vi "Try Add Sub Object.vi"(8 "error in":errorcluster, 10 "Sub Object":refnum<class "Sub Object.lvclass">, 11 "Object Dictionary in":refnum<class "Object Dictionary.lvclass">) -> (0 "error out":errorcluster, 1 "Success":bool, 3 "Object Dictionary out":refnum<class "Object Dictionary.lvclass">)   [LabVIEW 2020, in "CANopen.lvlib" / "Object Dictionary.lvclass"]
uses:
  Object Dictionary.lvclass
  Sub Object/Sub Object.lvclass
  Object Dictionary.lvclass/Object Dictionary.ctl
  Sub Objects Dictionary/Sub Objects Dictionary.lvclass
  Object Entry/Object Entry.lvclass
  Ordered-Dictionary/Ordered Object Dictionary/Source/Ordered Object Dictionary.lvclass
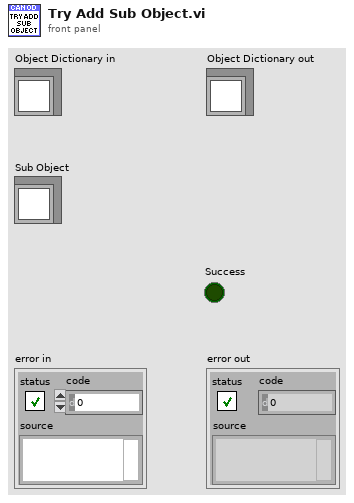
[diagram p1: front panel]
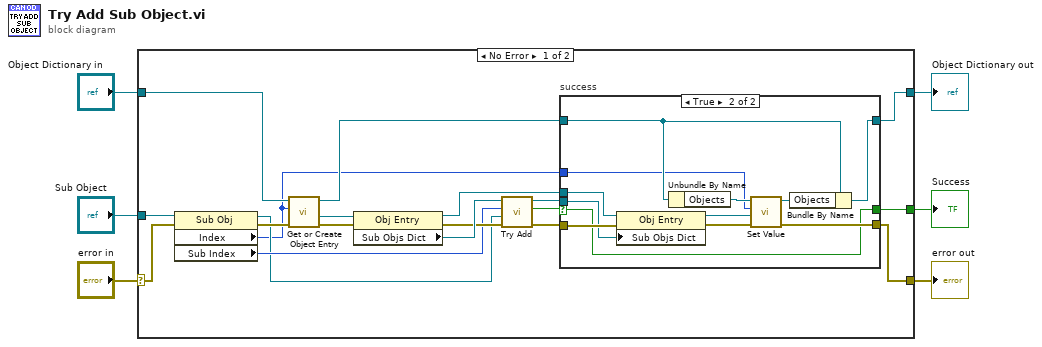
[diagram p0: block diagram]
diagram:
  n1 = case shown="No Error" "error in" {
    selector: "error in" -> [w24 w42]
    tunnel: [w17 w42] -> w5
    tunnel: [w18 w41] -> w3
    tunnel: "Object Dictionary in" -> [w12 w41]
    tunnel: "Sub Object" -> [w25 _]
    tunnel: [w15 _] -> w1
    frame No Error {
      n2 = property class="Sub Obj"(reference=w25, error in=w24) -> (reference out=w9:refnum<class "Sub Object.lvclass">, error out=w13:errorcluster, "Index"=w8:u16, "Sub Index"=w14:u8)
      n3 = call "Get or Create Object Entry.vi"("error in"=w13, "OD Index"=w8, "Obj Dict in"=w12) -> ("error out"=w10:errorcluster, "Obj Entry"=w7:refnum<class "Object Entry.lvclass">, "Obj Dict out"=w11:refnum<class "Object Dictionary.lvclass">)  [unwired: 6 in]
      n4 = property class="Obj Entry"(reference=w7, error in=w10) -> (reference out=w19:refnum<class "Object Entry.lvclass">, error out=w22:errorcluster, "Sub Objs Dict"=w23:refnum<class "Sub Objects Dictionary.lvclass">)
      n5 = call "Try Add.vi"("error in"=w22, "Sub Object"=w9, "Sub Index"=w14, "Sub Objects Dictionary in"=w23) -> ("error out"=w21:errorcluster, "Success"=w16:bool, "Sub Objects Dictionary out"=w20:refnum<class "Sub Objects Dictionary.lvclass">)  [unwired: 5 in]
      n6 = case "success" shown="True" w16 {
        selector: w16 -> [w27 w32]
        tunnel: w21 -> [w28 w40]
        tunnel: w20 -> [_ w39]
        tunnel: w19 -> [_ w38]
        tunnel: w11 -> [w26 w30]
        tunnel: [w26 w35] -> w18
        tunnel: [w28 w34] -> w17
        tunnel: [w27 w32] -> w15
        tunnel: w8 -> [_ w29]
        frame False {
        }
        frame True {
          n7 = property class="Obj Entry"(reference=w38, error in=w40, "Sub Objs Dict"=w39) -> (reference out=w33:refnum<class "Object Entry.lvclass">, error out=w36:errorcluster)
          n8 = Unbundle By Name(w30) -> ("Objects"=w31:refnum<class "Ordered Object Dictionary.lvclass">)
          n9 = call "Set Value.vi"("error in"=w36, "Value"=w33, "Key"=w29, "Ordered Object Dictionary in"=w31) -> ("error out"=w34:errorcluster, "Ordered Object Dictionary out"=w37:refnum<class "Ordered Object Dictionary.lvclass">)  [unwired: 6 in]
          n10 = Bundle By Name(cluster=w30, "Objects"=w37) -> (w35:refnum<class "Object Dictionary.lvclass">)
        }
      }
    }
    frame Error {
    }
  }
  "error out" <- w5
  "Object Dictionary out" <- w3
  "Success" <- w1
